vi "Lowpass Filter.vi"(6 "reset filter":bool, 8 "error in (no error)":errorcluster, 10 "Signal":cdb[](array[numeric]), 11 "Lock-in Detector in":refnum<class "Lock-in Detector.lvclass">) -> (0 "error out":errorcluster, 2 "Signal out":cdb[](array[numeric]), 3 "Lock-in Detector out":refnum<class "Lock-in Detector.lvclass">)   [LabVIEW 2021, in "Lock-in Detector.lvclass"]
uses:
  Lock-in Detector.lvclass
  Lock-in Detector.lvclass/Lock-in Detector.ctl
  Read End time.vi
  Read Time constant.vi
  Read Sample rate.vi
  Read Decimation factor.vi
  Write End time.vi
  Utilities/Fit/Smooth Background CDBL.vi
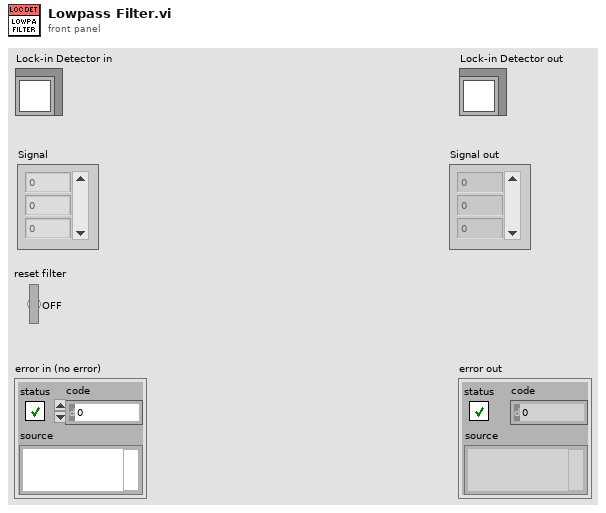
[diagram p1: front panel]
types:
  T1 = enum16{"Lowpass", "Highpass", "Bandpass", "Bandstop"}
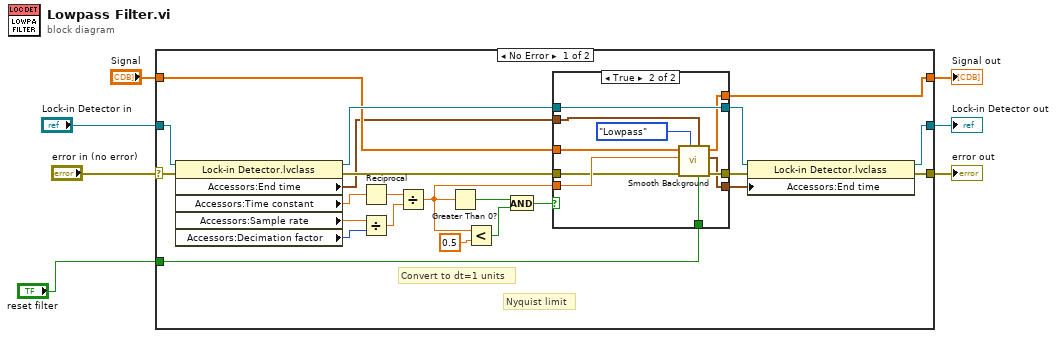
[diagram p0: block diagram]
diagram:
  n1 = case shown="No Error" "error in (no error)" {
    selector: "error in (no error)" -> [w23 w47]
    tunnel: [w12 w47] -> w6
    tunnel: [w10 w46] -> w4
    tunnel: "Lock-in Detector in" -> [w20 w46]
    tunnel: "Signal" -> [w16 w45]
    tunnel: [w15 w45] -> w2
    tunnel: "reset filter" -> [w8 _]
    frame No Error {
      # "Convert to dt=1 units"
      # "Nyquist limit"
      n2 = property class="Lock-in Detector.lvclass"(reference=w20, error in=w23) -> (reference out=w19:refnum<class "Lock-in Detector.lvclass">, error out=w21:errorcluster, "Accessors:End time"=w13:timestamp, "Accessors:Time constant"=w14:dbl, "Accessors:Sample rate"=w17:dbl, "Accessors:Decimation factor"=w18:i32)
      n3 = Reciprocal(x=w14) -> (1/x=w30:dbl)
      n4 = Divide(x=w17, y=w18) -> (x/y=w29:dbl)
      n5 = Divide(x=w30, y=w29) -> (x/y=w26:dbl)
      n6 = Greater Than 0?(x=w26) -> (x > 0?=w24:bool)
      n7 = Less?(x=w26, y=0.5) -> (x < y?=w27:bool)
      n8 = And(x=w24, y=w27) -> (x .and. y?=w25:bool)
      n9 = case shown="True" w25 {
        tunnel: w26 -> [_ w44]
        tunnel: w21 -> [w33 w43]
        tunnel: w19 -> [w34 w42]
        tunnel: [w34 w42] -> w11
        tunnel: [w33 w41] -> w22
        tunnel: w16 -> [w32 w39]
        tunnel: [w32 w38] -> w15
        tunnel: w13 -> [w31 w37]
        tunnel: [w31 w36] -> w9
        tunnel: w8 -> [_ w35]
        frame False {
        }
        frame True {
          n10 = call-poly "Smooth Background.vi"("reset filter"=w35, "t0"=w37, "Type"=T1."Lowpass", "Error In"=w43, "LP  F"=w44, "Data"=w39) -> ("Error Out"=w41:errorcluster, "End time"=w36:timestamp, "Data out"=w38:cdb[])  [unwired: 3 in]
        }
      }
      n11 = property class="Lock-in Detector.lvclass"(reference=w11, error in=w22, "Accessors:End time"=w9) -> (reference out=w10:refnum<class "Lock-in Detector.lvclass">, error out=w12:errorcluster)
    }
    frame Error {
    }
  }
  "error out" <- w6
  "Lock-in Detector out" <- w4
  "Signal out" <- w2
